vi "Save File DPT RMC Calculations.vi"(0 "Dryer IMC Data Input":T1={"Measured IMC (lbs)"=7.0, "Actual Initial RMC (%)"=7.0, "RMC (Desired %)"=100.0, "Bone Dry Wt(lbs)"=7.0, "Tolerance(%)"=5.0, "Actual Final RMC (%)"=7.0, "CEF (lbf/kWh)"=0.0, "Minimum Weight (lbf)"=0.0, "Average Weight (lbf)"=0.0, "Maximum Weight (lbf)"=0.0, "Measured IMC In Range?"=FALSE, "Moisture Reduction Factor"=55.5, "Field Use Factor"=1.04, "Empty Dryer Cold Weigth"=0.0, "Energy Standard"=enum."D2-Automatic Dryer", "Weight Cloth (lbs)"=0.0, "Relative Moisture Content (%)"=0.0, "Relative Moisture Content - Avg (%)"=0.0} {"Maximum Weight (lbf)" format="%03_6g"; "Average Weight (lbf)" format="%03_6g"; "Minimum Weight (lbf)" format="%03_6g"; "CEF (lbf/kWh)" format="%03_6g"; "Actual Final RMC (%)" format="%03_6g"; "Tolerance(%)" format="%0#_6g"; "Bone Dry Wt(lbs)" format="%03_6g"; "RMC (Desired %)" format="%0#_6g"; "Actual Initial RMC (%)" format="%03_6g"; "Measured IMC (lbs)" format="%0#_6g"}, 5 "Error In":errorcluster) -> (14 "Dryer IMC Data Output":T1={"Measured IMC (lbs)"=7.0, "Actual Initial RMC (%)"=7.0, "RMC (Desired %)"=100.0, "Bone Dry Wt(lbs)"=7.0, "Tolerance(%)"=5.0, "Actual Final RMC (%)"=7.0, "CEF (lbf/kWh)"=0.0, "Minimum Weight (lbf)"=0.0, "Average Weight (lbf)"=0.0, "Maximum Weight (lbf)"=0.0, "Measured IMC In Range?"=FALSE, "Moisture Reduction Factor"=55.5, "Field Use Factor"=1.04, "Empty Dryer Cold Weigth"=0.0, "Energy Standard"=enum."D2-Automatic Dryer", "Weight Cloth (lbs)"=0.0, "Relative Moisture Content (%)"=0.0, "Relative Moisture Content - Avg (%)"=0.0} {"Maximum Weight (lbf)" format="%03_6g"; "Average Weight (lbf)" format="%03_6g"; "Minimum Weight (lbf)" format="%03_6g"; "CEF (lbf/kWh)" format="%03_6g"; "Actual Final RMC (%)" format="%03_6g"; "Tolerance(%)" format="%0#_6g"; "Bone Dry Wt(lbs)" format="%03_6g"; "RMC (Desired %)" format="%0#_6g"; "Actual Initial RMC (%)" format="%03_6g"; "Measured IMC (lbs)" format="%0#_6g"}, 19 "Error Out":errorcluster)   [LabVIEW 2018, in "File Setup.lvlib"]
uses:
  File Setup.lvlib
  Type Definition/DPT IMC Data.ctl
  Washer DOE/Type Definitions/DOE Dryer Standard.ctl
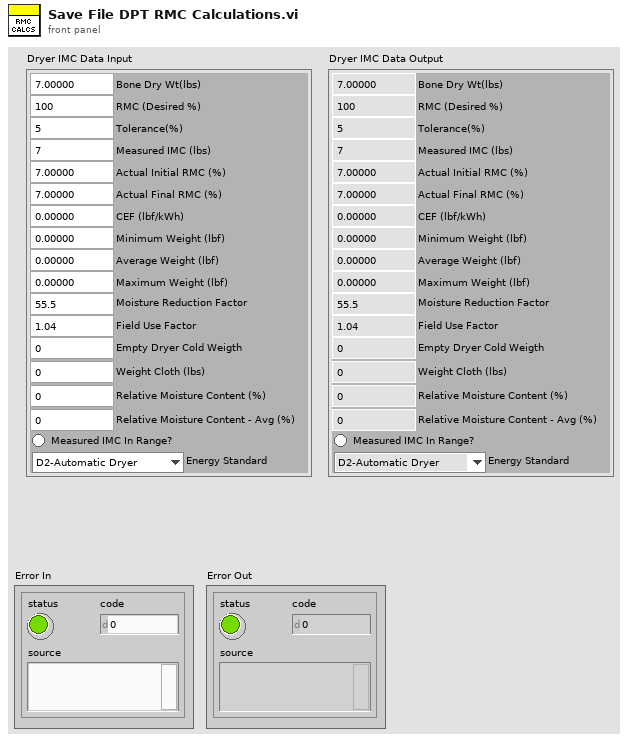
[diagram p1: front panel]
types:
  T1 = typedef "DPT IMC Data.ctl" = cluster{"Measured IMC (lbs)":dbl, "Actual Initial RMC (%)":dbl, "RMC (Desired %)":dbl, "Bone Dry Wt(lbs)":dbl, "Tolerance(%)":dbl, "Actual Final RMC (%)":dbl, "CEF (lbf/kWh)":dbl, "Minimum Weight (lbf)":dbl, "Average Weight (lbf)":dbl, "Maximum Weight (lbf)":dbl, "Measured IMC In Range?":bool, "Moisture Reduction Factor":dbl, "Field Use Factor":dbl, "Empty Dryer Cold Weigth":dbl, "Energy Standard":T2, "Weight Cloth (lbs)":dbl, "Relative Moisture Content (%)":dbl, "Relative Moisture Content - Avg (%)":dbl}
  T2 = typedef "DOE Dryer Standard.ctl" = enum16{"D2-Automatic Dryer", "D2-Timer Dryer", "D1-Automatic Dryer", "D1-Timer Dryer", "Other"}
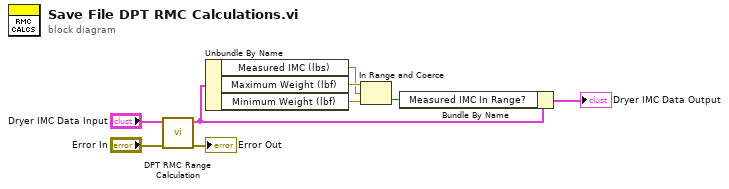
[diagram p0: block diagram]
diagram:
  n1 = call "DPT RMC Range Calculation.vi"("Error In"="Error In", "Dryer IMC Data Input"="Dryer IMC Data Input") -> ("Error Out"=→"Error Out":errorcluster, "Dryer IMC Data Output"=w3:T1)  [unwired: 8 in]
  n2 = Unbundle By Name(w3) -> ("Measured IMC (lbs)"=w4:dbl, "Maximum Weight (lbf)"=w6:dbl, "Minimum Weight (lbf)"=w5:dbl)
  n3 = In Range and Coerce(upper limit=w6, x=w4, lower limit=w5) -> (In Range?=w1:bool)  [unwired: 1 out]
  n4 = Bundle By Name(cluster=w3, "Measured IMC In Range?"=w1) -> (→"Dryer IMC Data Output":T1)
